vi "ConsoleFacade.vi"(0 "Data In":T4, 2 "Display State In":T2, 3 "Container State":T3) -> (6 "Data Out":T4, 7 "Display State Out":T2, 8 "Action":T1)   [LabVIEW 2016, in "ConsoleXControl.xctl"]
uses:
  ConsoleXControl.xctl
  <vilib>/_xctls/Action.ctl
  <vilib>/_xctls/XControlSupport.lvlib
  <vilib>/_xctls/Container State.ctl
  ConsoleData.ctl
  ConsoleState.ctl
panel:
  out "Console":string
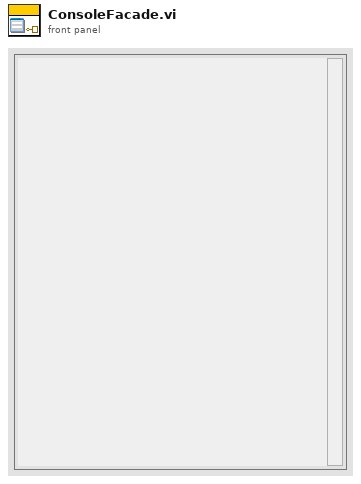
[diagram p1: front panel]
types:
  T1 = typedef "XControlSupport.lvlib/Action.ctl" = cluster{"Data Changed?":bool, "State Changed?":bool, "Action Name":string}
  T2 = typedef "ConsoleXControl.xctl/ConsoleState.ctl" = cluster{"Numeric":dbl}
  T3 = typedef "XControlSupport.lvlib/Container State.ctl" = cluster{"Indicator?":bool, "Run Mode?":bool, " Refnum":refnum<vi>}
  T4 = typedef "ConsoleXControl.xctl/ConsoleData.ctl" = string
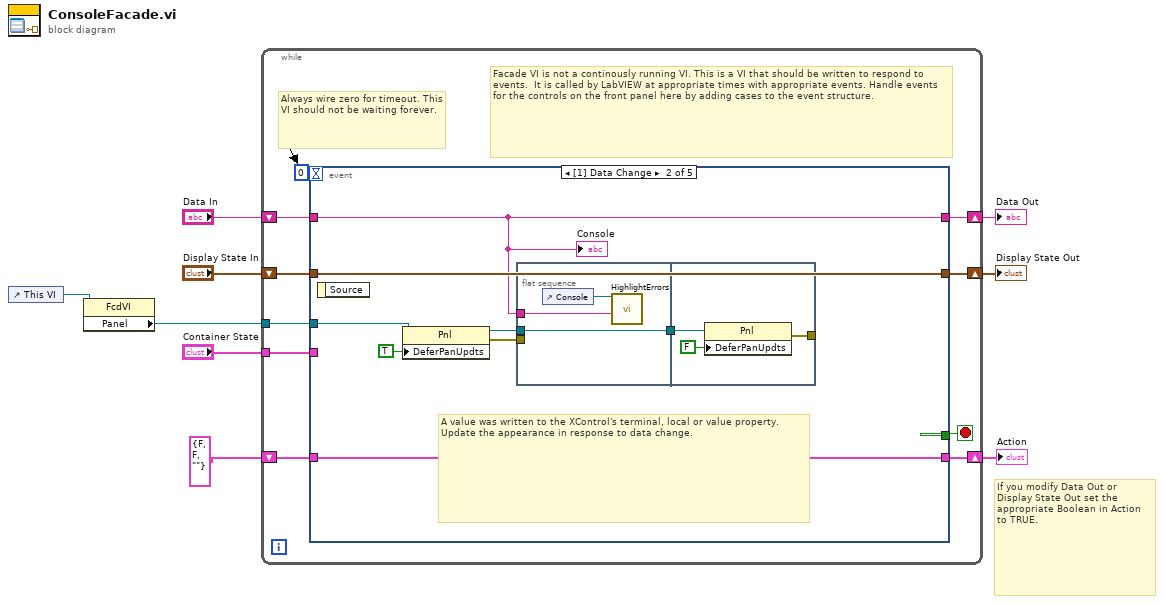
[diagram p0: block diagram]
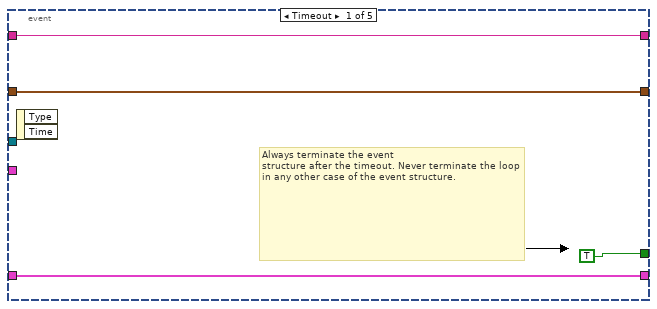
[diagram p2: hidden frame]
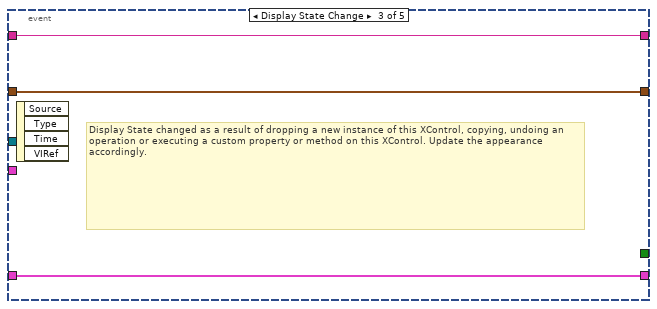
[diagram p3: hidden frame]
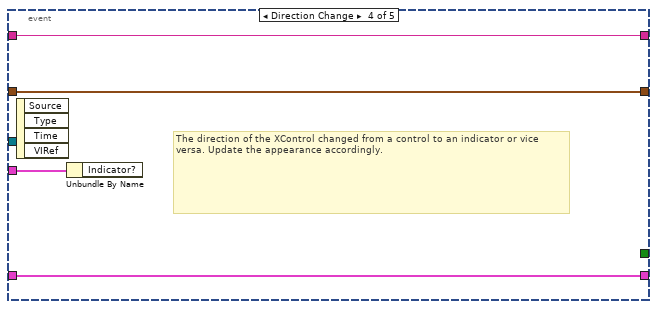
[diagram p4: hidden frame]
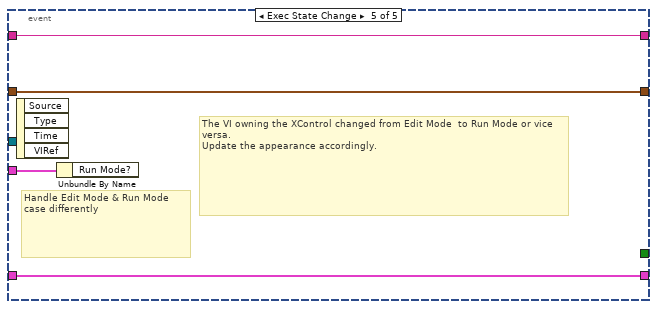
[diagram p5: hidden frame]
diagram:
  # "If you modify Data Out or\nDisplay State Out set the\nappropriate Boolean in Action\nto TRUE."
  n1 = control-ref of="This VI"() -> (w2:refnum<vi>)
  n2 = property class="FcdVI"(reference=w2) -> ("Panel"=w1:refnum<vi>)  [unwired: 1 in, 2 out]
  n3 = while {
    shift-right: [w18] -> w6
    shift-left: "Display State In" -> [w19]
    tunnel: "Container State" -> [w15]
    shift-right: [w13] -> w9
    shift-left: "Data In" -> [w14]
    shift-right: [w11] -> w4
    shift-left: T1 {"Data Changed?"=FALSE, "State Changed?"=FALSE, "Action Name"=""} ("Action") -> [w12]
    tunnel: w1 -> [w10]
    stop <- w17 stop-if-true
    # "Facade VI is not a continously running VI. This is a VI that should be written to respond to events.  It is called by LabVIEW at appropriate times with appropriate events. Handle events for the controls on the front panel here by adding cases to the event structure."
    # "Always wire zero for timeout. This\nVI should not be waiting forever."
    n4 = event shown="[1] Data Change" {
      selector: _ -> [_ _ _ _ _]
      dyn-events: _ -> [_ _ _ _ _]
      timeout: 0 -> [_ _ _ _ _]
      tunnel: w19 -> [w21 w31 w40 w43 w47]
      tunnel: [w21 w31 w40 w43 w47] -> w18
      tunnel: [TRUE _ _ _ _] -> w17
      tunnel: w15 -> [_ _ _ w44 w48]
      tunnel: w14 -> [w20 w29 w39 w42 w46]
      tunnel: [w20 w29 w39 w42 w46] -> w13
      tunnel: [w22 w30 w38 w41 w45] -> w11
      tunnel: w12 -> [w22 w30 w38 w41 w45]
      tunnel: w10 -> [_ w27 _ _ _]
      event Timeout {
        # "Always terminate the event\nstructure after the timeout. Never terminate the loop in any other case of the event structure."
        n5 = event-data() -> ()  [unwired: 1 in, 2 out]
      }
      event Data Change {
        # "A value was written to the XControl's terminal, local or value property.\nUpdate the appearance in response to data change."
        n6 = event-data() -> ()  [unwired: 1 in, 1 out]
        n7 = property class="Pnl"(reference=w27, "DeferPanUpdts"=TRUE ("Defer Panel Updates")) -> (reference out=w25:refnum<vi>, error out=w24:errorcluster)  [unwired: 1 in]
        n8 = flat-sequence {
          tunnel: w29 -> [w34]
          tunnel: [w32] -> w26
          tunnel: w25 -> [w32]
          tunnel: w24 -> [_]
          tunnel: w26 -> [w36]
          tunnel: [w35] -> _
          frame #0 {
            n9 = control-ref of="Console"() -> (w33:refnum<vi>)
            n10 = call "HighlightErrors.vi"("String"=w34, "Console"=w33) -> ()  [unwired: 10 in]
          }
          frame #1 {
            n11 = property class="Pnl"(reference=w36, "DeferPanUpdts"=FALSE ("Defer Panel Updates")) -> (error out=w35:errorcluster)  [unwired: 1 in, 1 out]
          }
        }
        "Console" <- w29
      }
      event Display State Change {
        # "Display State changed as a result of dropping a new instance of this XControl, copying, undoing an operation or executing a custom property or method on this XControl. Update the appearance accordingly."
        n12 = event-data() -> ()  [unwired: 1 in, 4 out]
      }
      event Direction Change {
        # "The direction of the XControl changed from a control to an indicator or vice versa. Update the appearance accordingly."
        n13 = event-data() -> ()  [unwired: 1 in, 4 out]
        n14 = Unbundle By Name(w44) -> ()  [unwired: 1 out]
      }
      event Exec State Change {
        # "The VI owning the XControl changed from Edit Mode  to Run Mode or vice versa.\nUpdate the appearance accordingly."
        # "Handle Edit Mode & Run Mode\ncase differently"
        n15 = event-data() -> ()  [unwired: 1 in, 4 out]
        n16 = Unbundle By Name(w48) -> ()  [unwired: 1 out]
      }
    }
  }
  "Display State Out" <- w6
  "Data Out" <- w9
  "Action" <- w4
